vi "test Get Chamber Status-Error Before Get Status.vi"(8 "error in (no error)":errorcluster, 11 "TestCase in":refnum<class "Get Chamber Status.lvclass">) -> (0 "error out":errorcluster, 3 "TestCase out":refnum<class "Get Chamber Status.lvclass">)   [LabVIEW 2018, in "Get Chamber Status.lvclass"]
uses:
  Get Chamber Status.lvclass
  Libraries/Thermal Chamber Response Simulator/Thermal Chamber Response Simulator.lvlib
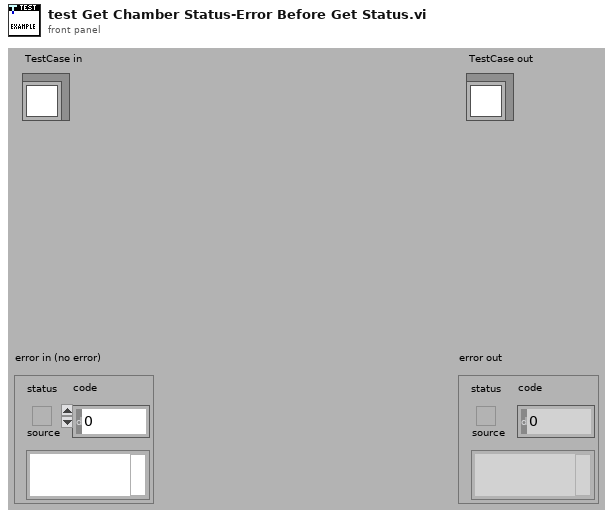
[diagram p1: front panel]
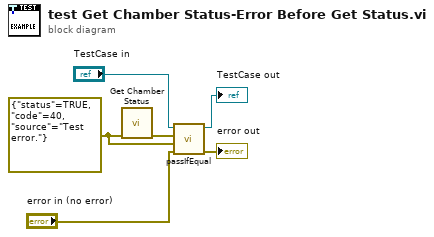
[diagram p0: block diagram]
diagram:
  w5 = errorcluster {"status"=TRUE, "code"=40, "source"="Test error."} ("Test Error")
  n1 = call "Get Chamber Status.vi"("error in (no error)"=w5) -> ("error out"=w6:errorcluster)  [unwired: 5 in, 5 out]
  n2 = call-dynamic "passIfEqual.vi"("error in (no error)"="error in (no error)", "y"=w5, "x"=w6, "TestCase in"="TestCase in") -> ("error out"=→"error out":errorcluster, "TestCase out"=→"TestCase out":refnum<class "Get Chamber Status.lvclass">)  [unwired: 6 in]
